vi "clFile_readFromFile.vi"(10 "file (use dialog)":path) -> (2 "clFileReader.lvclass":refnum<class "clFileReader.lvclass">, 3 "clFile.lvclass":refnum<class "clFile.lvclass">)   [LabVIEW 2016, in "vi_lib.lvlib" / "clFile.lvclass"]
uses:
  clFile.lvclass
  clFileReader/clFileReader.lvclass
  clFile.lvclass/clFile.ctl
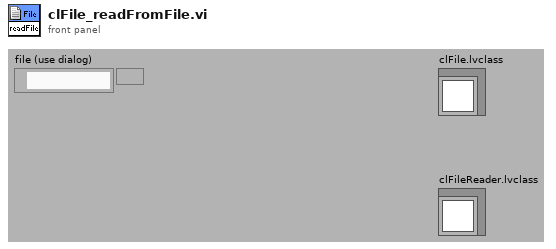
[diagram p1: front panel]
types:
  T1 = enum16{"open", "replace", "create", "open or create", "replace or create", "replace or create with confirmation"}
  T2 = enum16{"deny read/write", "deny write-only", "deny none"}
  T3 = enum16{"big-endian, network order", "native, host order", "little-endian"}
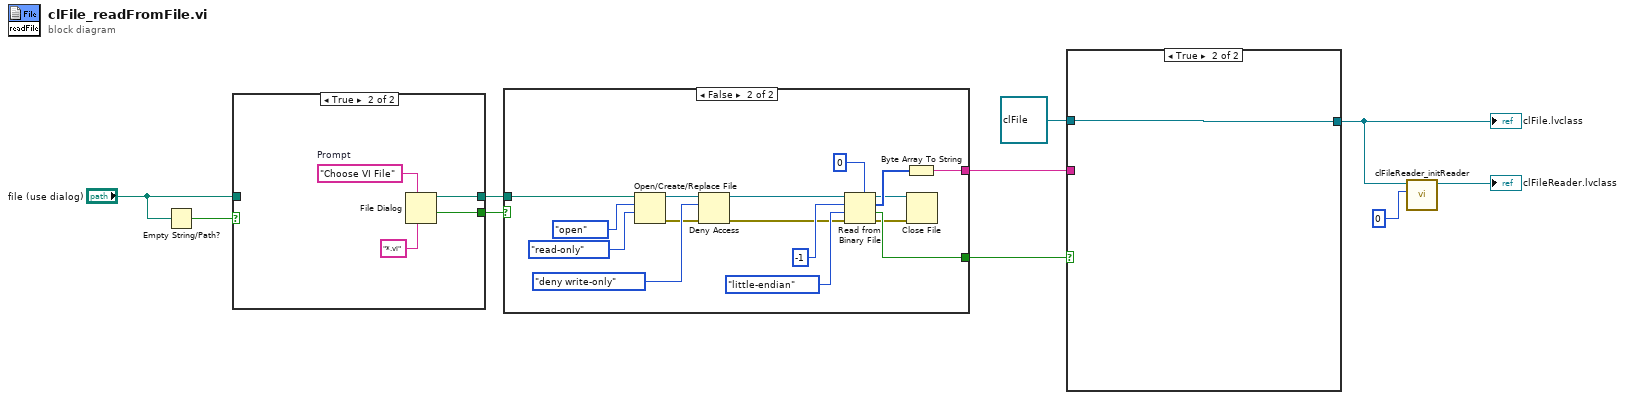
[diagram p0: block diagram]
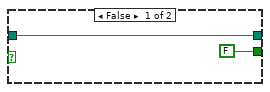
[diagram p2: hidden frame]
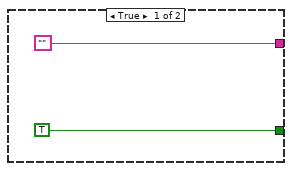
[diagram p3: hidden frame]
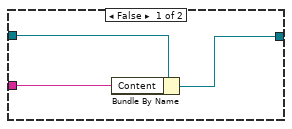
[diagram p4: hidden frame]
diagram:
  n1 = Empty String/Path?(string/path="file (use dialog)") -> (empty?=w1:bool)
  n2 = case shown="True" w1 {
    tunnel: [w12 w15] -> w8
    tunnel: "file (use dialog)" -> [w12 _]
    tunnel: [FALSE ("cancelled") w14] -> w7
    frame False {
    }
    frame True {
      w13 = "Choose VI File"  # Prompt
      n3 = File Dialog(6:"*.vi" ("pattern (all files)"), 7:w13) -> (1:w14:bool, 3:w15:path)  [unwired: 1 in, 6 out]
    }
  }
  n4 = case shown="False" w7 {
    tunnel: [TRUE ("cancelled") w26] -> w10
    tunnel: ["" w22] -> w9
    tunnel: w8 -> [_ w21]
    frame True {
    }
    frame False {
      n5 = Open/Create/Replace File(file path (use dialog)=w21, operation (0:open)=T1."open", access (0:read/write)=enum16{"read/write", "read-only", "write-only"}."read-only") -> (refnum out=w30:refnum<file>, error out=w29:errorcluster)  [unwired: 1 in, 3 out]
      n6 = Deny Access(4:w29, 6:T2."deny write-only" ("deny mode (0:deny read/write)"), 7:w30) -> (0:w25:errorcluster, 3:w33:refnum<file>)
      n7 = Read from Binary File(5:u8 0, 8:w25, 9:T3."little-endian" ("Byte Order"), 10:-1 ("Data Size (in bytes)"), 11:w33) -> (0:w19:errorcluster, 1:w26:bool, 2:w23:u8[], 3:w20:refnum<file>)  [unwired: 1 out]
      n8 = Byte Array To String(unsigned byte array=w23) -> (string=w22:string)
      n9 = Close File(refnum=w20, error in=w19) -> ()  [unwired: 2 out]
    }
  }
  n10 = case shown="True" w10 {
    tunnel: w9 -> [w37 _]
    tunnel: refnum<class "clFile.lvclass"> refnum ("clFile.lvclass") -> [w36 w38]
    tunnel: [w35 w38] -> w5
    frame False {
      n11 = Bundle By Name(cluster=w36, "Content"=w37) -> (w35:refnum<class "clFile.lvclass">)
    }
    frame True {
    }
  }
  "clFile.lvclass" <- w5
  n12 = call "clFileReader_initReader.vi"("HiddenOffset"=u32 0, "clFile.lvclass"=w5) -> ("clFileReader.lvclass"=→"clFileReader.lvclass":refnum<class "clFileReader.lvclass">)  [unwired: 1 in, 8 out]
